vi "rid.set.vi"(8 "error in (no error)":errorcluster, 10 "rid":string, 11 "workspace in":refnum<class "workspace.lvclass">) -> (0 "error out":errorcluster, 3 "workspace out":refnum<class "workspace.lvclass">)   [LabVIEW 2020, in "nominal types.lvlib" / "workspace.lvclass"]
uses:
  workspace.lvclass
  workspace.lvclass/workspace.ctl
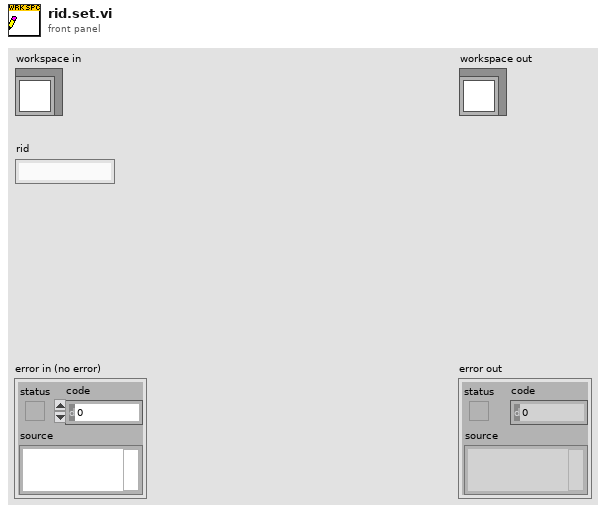
[diagram p1: front panel]
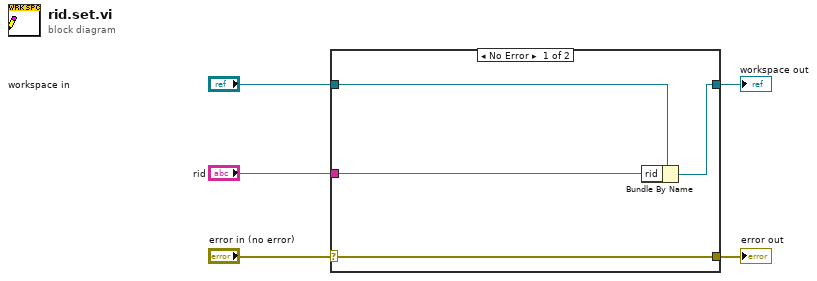
[diagram p0: block diagram]
diagram:
  n1 = case shown="No Error" "error in (no error)" {
    selector: "error in (no error)" -> [w9 w10]
    tunnel: [w9 w10] -> w4
    tunnel: [w7 w11] -> w2
    tunnel: "workspace in" -> [w8 w11]
    tunnel: "rid" -> [w6 _]
    frame No Error {
      n2 = Bundle By Name(cluster=w8, "rid"=w6) -> (w7:refnum<class "workspace.lvclass">)
    }
    frame Error {
    }
  }
  "error out" <- w4
  "workspace out" <- w2
